vi "浮标电源管理UI.vi"() -> ()   [LabVIEW 2016, in "环境动力监测库.lvlib" / "浮标电源管理.lvlib"]
uses:
  <vilib>/Utility/miscctls.llb/LVPointTypeDef.ctl
  <vilib>/Utility/config.llb/NI_LVConfig.lvlib
  <vilib>/ptbypt/NI_PtbyPt.lvlib
panel:
  in  "控制对象":enum16{"所有辅助设备", "气象电源", "视频电源"}(ring)=enum."视频电源"
  in  "辅助电源控制类型":enum16{"定时控制", "电压控制"}(ring)
  in  "辅助设备电源关闭时间":u16(ring)=12 items=["00H", "01H", "02H", "03H", "04H", "05H", "06H", "07H", "08H", "09H", "10H", "11H", "12H", "13H", "14H", "15H", "16H", "17H", "18H", "19H", "20H", "21H", "22H", "23H"]
  in  "辅助设备电源开启时间":u16(ring)=12 items=["00H", "01H", "02H", "03H", "04H", "05H", "06H", "07H", "08H", "09H", "10H", "11H", "12H", "13H", "14H", "15H", "16H", "17H", "18H", "19H", "20H", "21H", "22H", "23H"]
  in  "开启辅助电源控制":bool
  in  "辅助设备电源开启电压 V":dbl=13.0
  in  "辅助设备电源关闭电压 V":dbl=12.0
  in  "视频电源":bool
  in  "气象电源":bool
  in  "总磷总氮电源":bool
  in  "氨氮电源":bool
  in  "多参数电源":bool
  in  "IO模块启用":bool
  in  "IO串口":refnum<visa-resource-name>
  in  "串口启用":bool
  out "电压报警":bool
  in  "低压报警解除阈值 V":dbl=50.0
  in  "低压报警阈值 V":dbl=50.0
  out "当前电压":dbl=21.0 format="%.2f V"
  out "通讯状态":bool
  # "仪器电源管理"
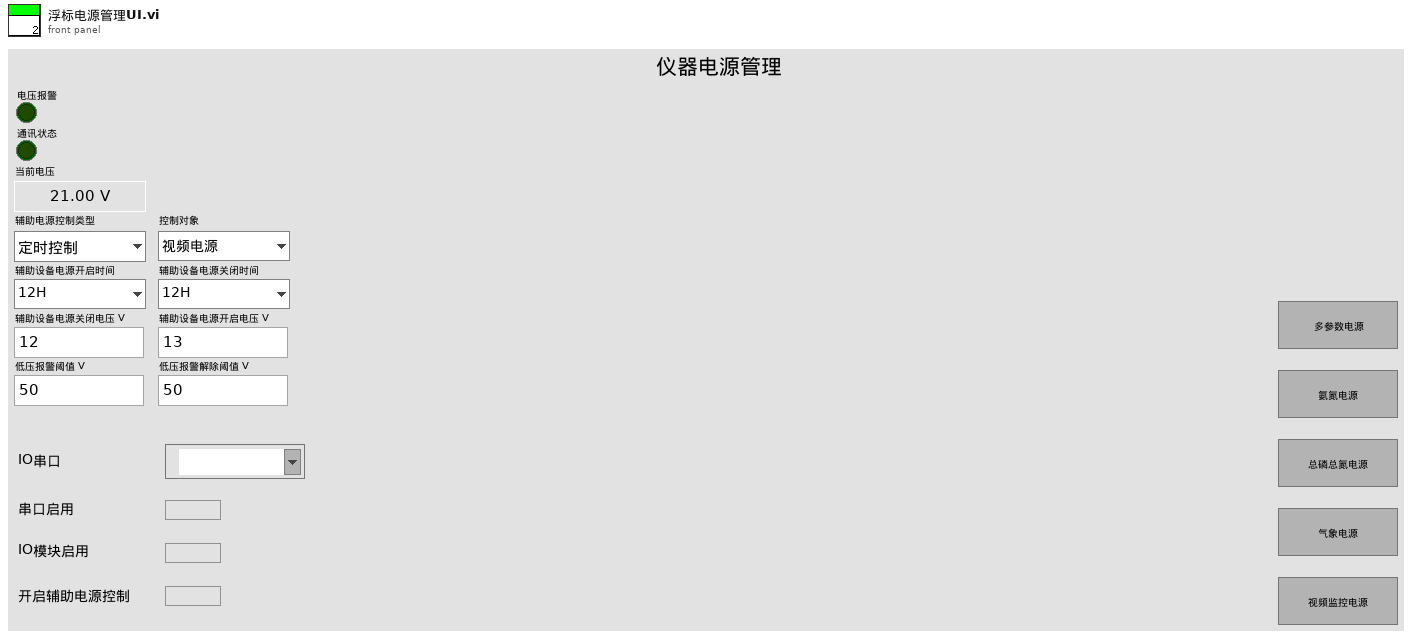
[diagram p1: front panel]
types:
  T1 = typedef "LVPointTypeDef.ctl" = cluster{"Horizontal":i16, "Vertical":i16}
  T2 = cluster{"AD0":dbl, "AD1":dbl, "AD2":dbl, "AD3":dbl, "AD4":dbl, "AD5":dbl, "AD6":dbl, "AD7":dbl}
  T3 = cluster{"低压报警阈值 V":dbl, "低压报警解除阈值 V":dbl, "高温报警阈值 ℃":dbl, "高温报警解除阈值 ℃":dbl, "湿度报警阈值 %":dbl, "湿度报警解除阈值 %":dbl}
  T4 = typedef "LVDateTimeRec.ctl" = cluster{"秒数的小数部分":dbl, "秒":i32, "分":i32, "时":i32, "日":i32, "月":i32, "年":i32, "天数（周）":i32, "天数（年）":i32, "DST":i32}
  T5 = cluster{"时间标识":timestamp, "设备":string, "报警信息":string}
  T6 = typedef "NI_LVConfig.lvlib/Config Data RefNum.ctl" = refnum<k1>
  T7 = enum8{"Enabled", "Disabled", "Disabled and Grayed Out"}
  T8 = cluster{"Registers[0]":u16, "Registers[1]":u16, "Registers[2]":u16, "Registers[3]":u16, "Registers[4]":u16, "Registers[5]":u16, "Registers[6]":u16, "Registers[7]":u16}
  T9 = cluster{"网络状态":bool, "电源管理":cluster{"电源管理":bool, "氨氮电源":bool, "总磷电源":bool, "总氮电源":bool, "多参数电源":bool, "CODMn电源":bool, "CODCr电源":bool, "灯带电源":bool, "照明电源":bool}, "北斗-GPS":cluster{"北斗":cluster{"经度:":sgl, "纬度:":sgl, "北斗监测":bool}, "GPS":cluster{"经度:":sgl, "纬度: ":sgl, "GPS监测":bool}}}
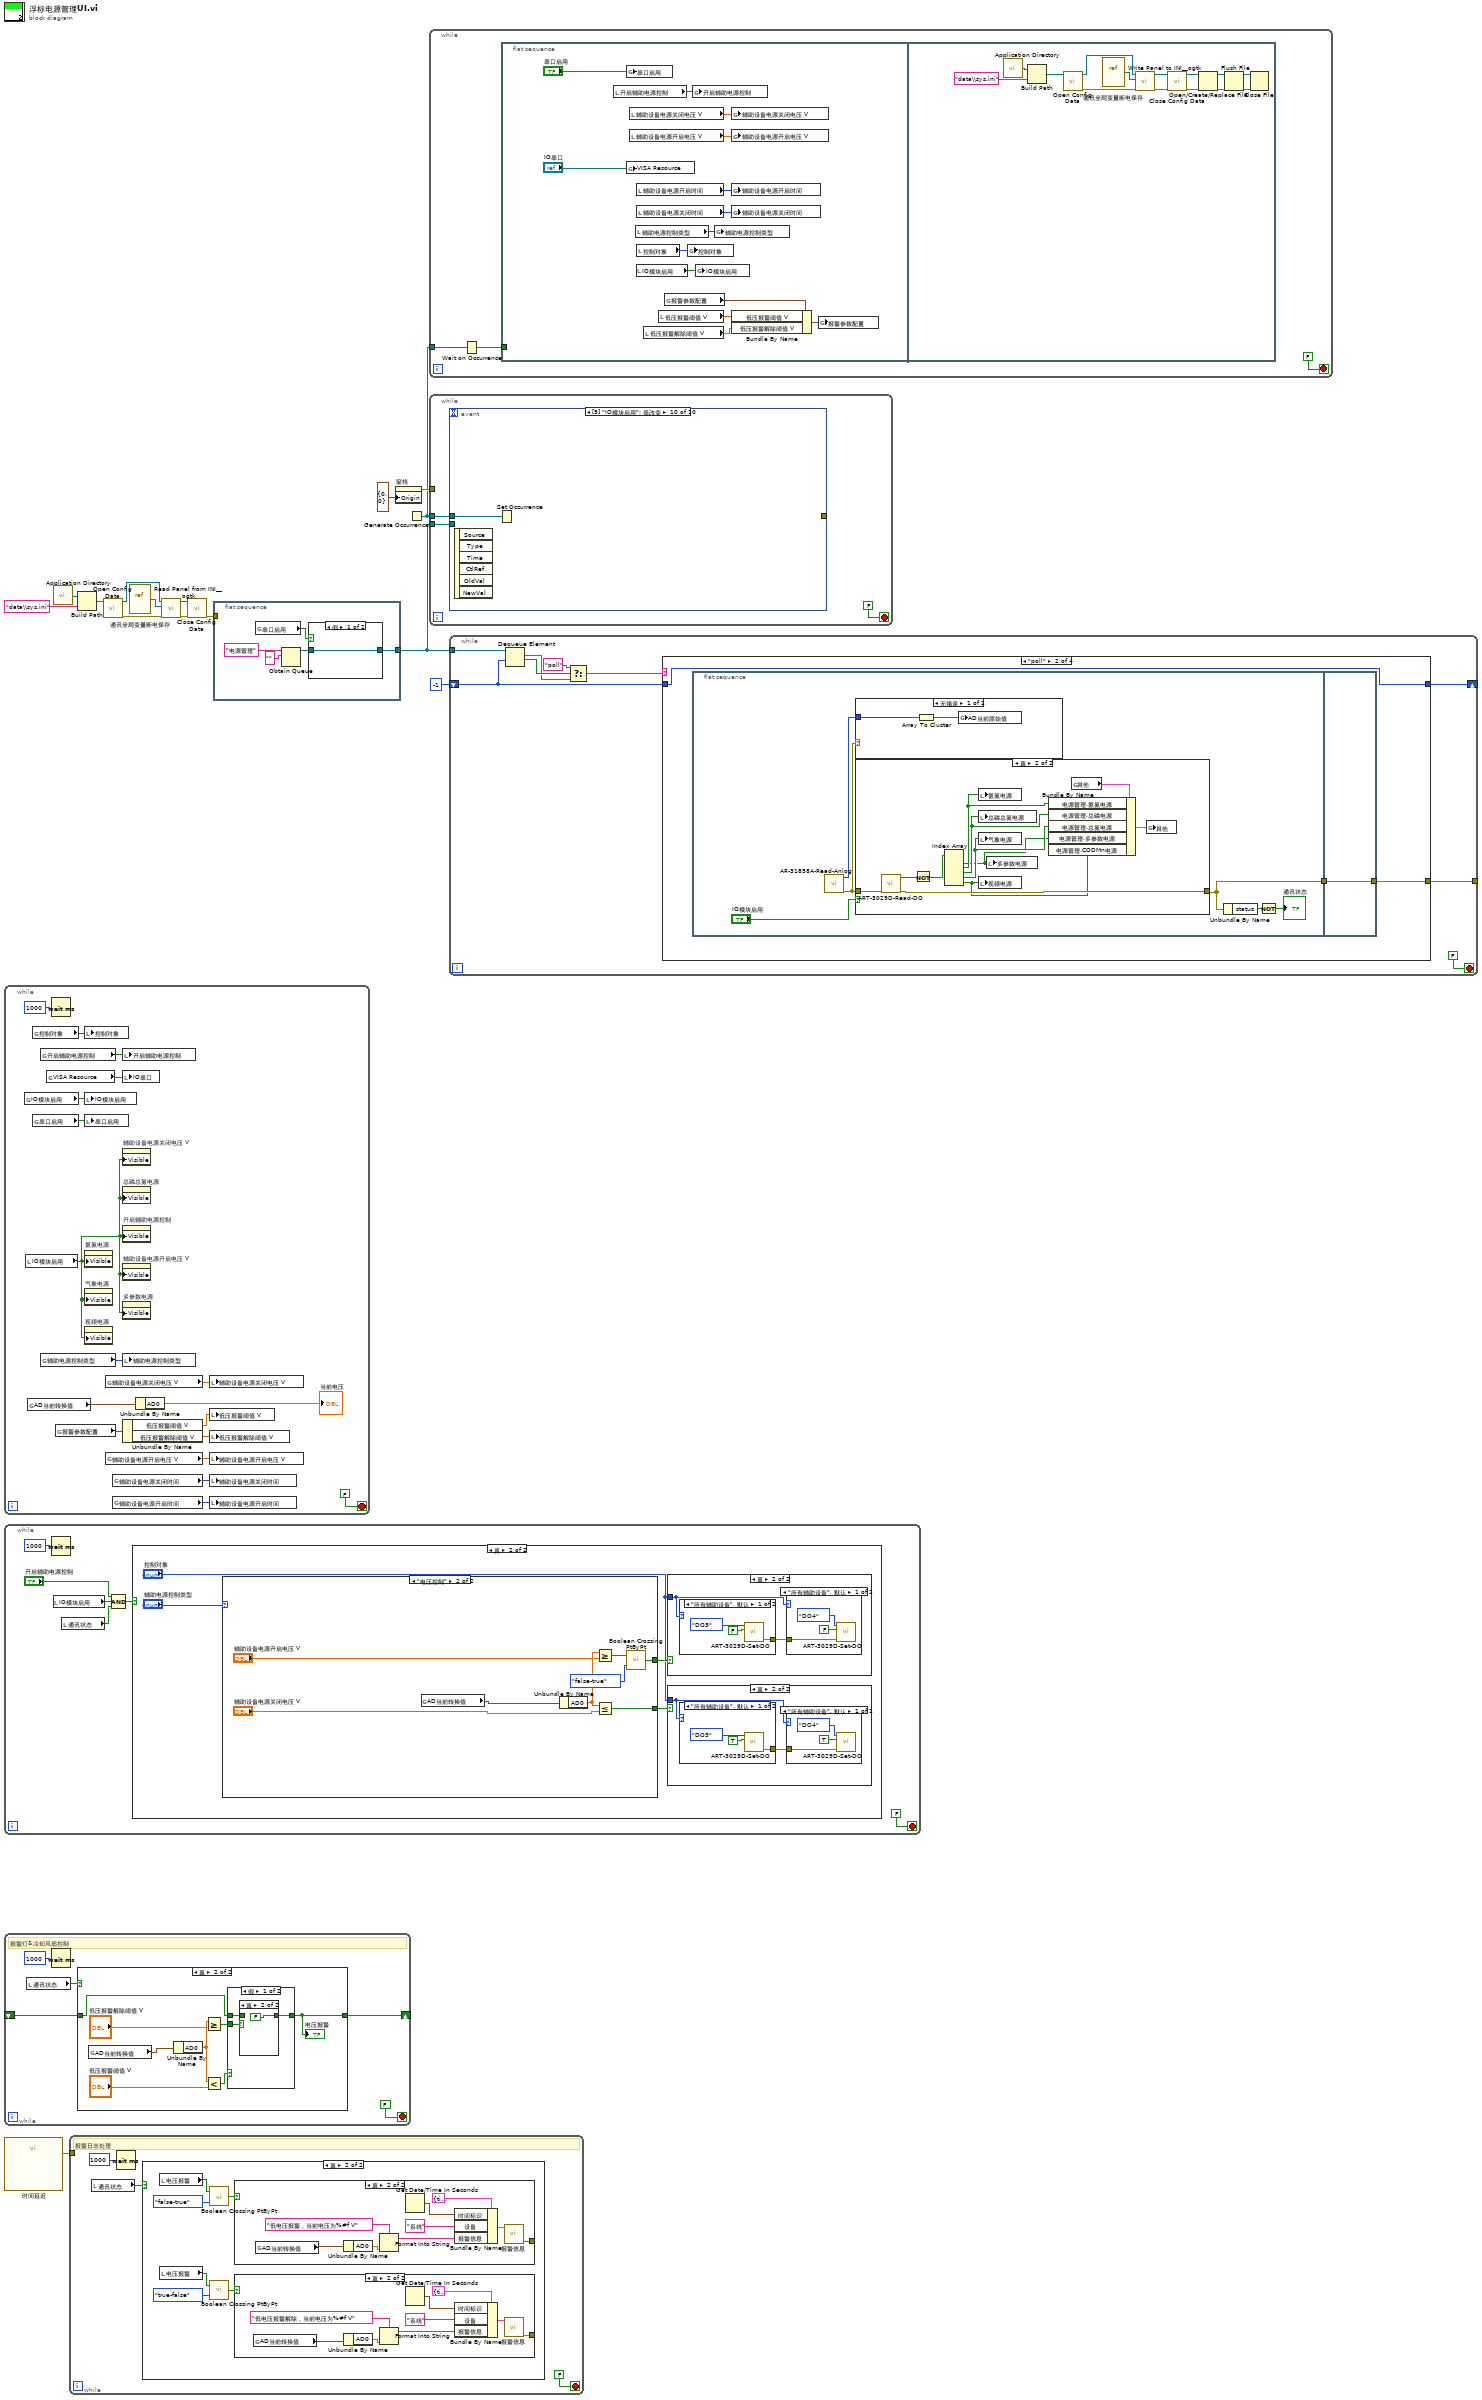
[diagram p0: block diagram]
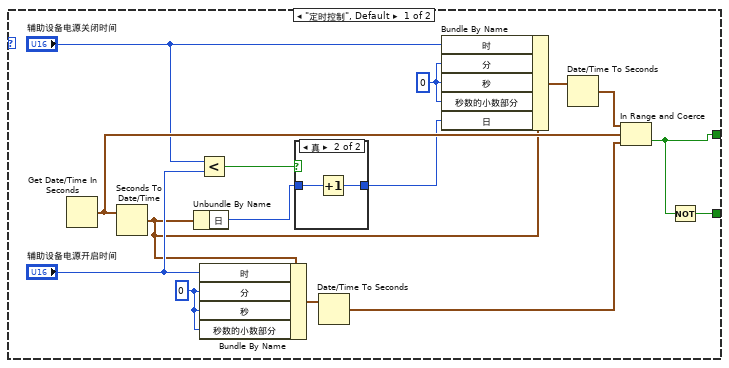
[diagram p6: hidden frame]
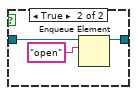
[diagram p11: hidden frame]
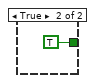
[diagram p17: hidden frame]
diagram:
  n1 = while {
    stop <- FALSE stop-if-true
    n2 = global read "通讯全局变量断电保存.vi" "IO模块启用"() -> (w25:bool)
    n3 = local read "IO模块启用"() -> (w22:bool)
    n4 = global read "断电保存全局变量.vi" "AD当前转换值"() -> (w16:T2)
    n5 = global read "通讯全局变量断电保存.vi" "控制对象"() -> (w17:enum16{"所有辅助设备", "气象电源", "视频电源"})
    n6 = global read "通讯全局变量断电保存.vi" "串口启用"() -> (w27:bool)
    n7 = global read "通讯全局变量断电保存.vi" "开启辅助电源控制"() -> (w21:bool)
    n8 = global read "通讯全局变量断电保存.vi" "辅助电源控制类型"() -> (w20:enum16{"定时控制", "电压控制"})
    n9 = global read "通讯全局变量断电保存.vi" "VISA Resource"() -> (w26:refnum<visa-resource-name>)
    n10 = Wait (ms)(milliseconds to wait=u32 1000 ("等待时间（毫秒）")) -> ()  [unwired: 1 out]
    n11 = global read "通讯全局变量断电保存.vi" "报警参数配置"() -> (w32:T3)
    n12 = local write "控制对象"(w17) -> ()
    n13 = local write "IO模块启用"(w25) -> ()
    n14 = local write "串口启用"(w27) -> ()
    n15 = property on="氨氮电源" class="Bool (严格)"("Visible"=w22) -> ()  [unwired: 2 in, 2 out]
    n16 = property on="气象电源" class="Bool (严格)"("Visible"=w22) -> ()  [unwired: 2 in, 2 out]
    n17 = property on="视频电源" class="Bool (严格)"("Visible"=w22) -> ()  [unwired: 2 in, 2 out]
    n18 = global read "通讯全局变量断电保存.vi" "辅助设备电源关闭电压 V"() -> (w24:dbl)
    n19 = global read "通讯全局变量断电保存.vi" "辅助设备电源开启电压 V"() -> (w23:dbl)
    n20 = global read "通讯全局变量断电保存.vi" "辅助设备电源关闭时间"() -> (w19:u16)
    n21 = global read "通讯全局变量断电保存.vi" "辅助设备电源开启时间"() -> (w18:u16)
    n22 = local write "开启辅助电源控制"(w21) -> ()
    n23 = local write "IO串口"(w26) -> ()
    n24 = property on="辅助设备电源关闭电压 V" class="DigNum (严格)"("Visible"=w22) -> ()  [unwired: 2 in, 2 out]
    n25 = property on="总磷总氮电源" class="Bool (严格)"("Visible"=w22) -> ()  [unwired: 2 in, 2 out]
    n26 = property on="开启辅助电源控制" class="Bool (严格)"("Visible"=w22) -> ()  [unwired: 2 in, 2 out]
    n27 = property on="辅助设备电源开启电压 V" class="DigNum (严格)"("Visible"=w22) -> ()  [unwired: 2 in, 2 out]
    n28 = property on="多参数电源" class="Bool (严格)"("Visible"=w22) -> ()  [unwired: 2 in, 2 out]
    n29 = local write "辅助电源控制类型"(w20) -> ()
    n30 = Unbundle By Name(w32) -> ("低压报警阈值 V"=w30:dbl, "低压报警解除阈值 V"=w29:dbl)
    n31 = Unbundle By Name(w16) -> ("AD0"=→"当前电压":dbl)
    n32 = local write "辅助设备电源关闭电压 V"(w24) -> ()
    n33 = local write "低压报警阈值 V"(w30) -> ()
    n34 = local write "低压报警解除阈值 V"(w29) -> ()
    n35 = local write "辅助设备电源开启电压 V"(w23) -> ()
    n36 = local write "辅助设备电源关闭时间"(w19) -> ()
    n37 = local write "辅助设备电源开启时间"(w18) -> ()
  }
  n38 = while {
    stop <- FALSE stop-if-true
    n39 = Wait (ms)(milliseconds to wait=u32 1000 ("等待时间（毫秒）")) -> ()  [unwired: 1 out]
    n40 = local read "IO模块启用"() -> (w36:bool)
    n41 = local read "通讯状态"() -> (w37:bool)
    n42 = Compound Arithmetic op=AND ("复合运算")("开启辅助电源控制", w36, w37) -> (w34:bool)
    n43 = case shown="真" w34 {
      frame False {
      }
      frame True {
        n44 = case shown="\"电压控制\"" "辅助电源控制类型" {
          tunnel: [w53 w72] -> w41
          tunnel: [w52 w71] -> w43
          frame "定时控制", Default {
            w55 = 0
            w54 = 0
            n45 = Get Date/Time In Seconds() -> (seconds since 1Jan1904=w66:timestamp)
            n46 = Seconds To Date/Time(time stamp (now)=w66) -> (date time rec=w60:T4)  [unwired: 1 in]
            n47 = Unbundle By Name(w60) -> ("日"=w61:i32)
            n48 = Less?(x="辅助设备电源关闭时间", y="辅助设备电源开启时间") -> (x < y?=w63:bool)
            n49 = Bundle By Name(cluster=w60, "时"="辅助设备电源开启时间", "分"=w54, "秒"=w54, "秒数的小数部分"=w54) -> (w56:T4)
            n50 = case shown="真" w63 {
              tunnel: w61 -> [w67 w69]
              tunnel: [w67 w68] -> w62
              frame False {
              }
              frame True {
                n51 = Increment(x=w69) -> (x+1=w68:i32)
              }
            }
            n52 = Date/Time To Seconds(2:w56) -> (0:w59:timestamp)  [unwired: 1 in]
            n53 = Bundle By Name(cluster=w60, "时"="辅助设备电源关闭时间", "分"=w55, "秒"=w55, "秒数的小数部分"=w55, "日"=w62) -> (w57:T4)
            n54 = Date/Time To Seconds(2:w57) -> (0:w58:timestamp)  [unwired: 1 in]
            n55 = In Range and Coerce(upper limit=w58, x=w66, lower limit=w59) -> (In Range?=w53:bool)  [unwired: 1 out]
            n56 = Not(x=w53) -> (.not. x?=w52:bool)
          }
          frame "电压控制" {
            n57 = global read "断电保存全局变量.vi" "AD当前转换值"() -> (w70:T2)
            n58 = Unbundle By Name(w70) -> ("AD0"=w76:dbl)
            n59 = Greater Or Equal?(x=w76, y="辅助设备电源开启电压 V") -> (x >= y?=w73:bool)
            n60 = Less Or Equal?(x=w76, y="辅助设备电源关闭电压 V") -> (x <= y?=w71:bool)
            n61 = call <vilib>:"Boolean Crossing PtByPt.vi"("direction"=enum16{"either", "false-true", "true-false"}."false-true", "input"=w73) -> ("crossing"=w72:bool)  [unwired: 1 in]
          }
        }
        n62 = case shown="真" w41 {
          tunnel: "控制对象" -> [_ w44]
          frame False {
          }
          frame True {
            n63 = case shown="\"所有辅助设备\", 默认" w44 {
              tunnel: [w50 _] -> w45
              frame "所有辅助设备", Default {
                n64 = call "ART-3029D-Set-DO.vi"("value"=FALSE, "DI"=enum16{"DO0", "DO1", "DO2", "DO3", "DO4"}."DO3") -> ("error out"=w50:errorcluster)  [unwired: 9 in]
              }
              frame "视频电源" {
              }
            }
            n65 = case shown="\"所有辅助设备\", 默认" w44 {
              tunnel: w45 -> [w48 _]
              frame "所有辅助设备", Default {
                n66 = call "ART-3029D-Set-DO.vi"("error in (no error)"=w48, "value"=FALSE, "DI"=enum16{"DO0", "DO1", "DO2", "DO3", "DO4"}."DO4") -> ()  [unwired: 8 in, 1 out]
              }
              frame "气象电源" {
              }
            }
          }
        }
        n67 = case shown="真" w43 {
          tunnel: "控制对象" -> [_ w78]
          frame False {
          }
          frame True {
            n68 = case shown="\"所有辅助设备\", 默认" w78 {
              tunnel: [w84 _] -> w79
              frame "所有辅助设备", Default {
                n69 = call "ART-3029D-Set-DO.vi"("value"=TRUE, "DI"=enum16{"DO0", "DO1", "DO2", "DO3", "DO4"}."DO3") -> ("error out"=w84:errorcluster)  [unwired: 9 in]
              }
              frame "视频电源" {
              }
            }
            n70 = case shown="\"所有辅助设备\", 默认" w78 {
              tunnel: w79 -> [w82 _]
              frame "所有辅助设备", Default {
                n71 = call "ART-3029D-Set-DO.vi"("error in (no error)"=w82, "value"=TRUE, "DI"=enum16{"DO0", "DO1", "DO2", "DO3", "DO4"}."DO4") -> ()  [unwired: 8 in, 1 out]
              }
              frame "气象电源" {
              }
            }
          }
        }
      }
    }
  }
  n72 = while {
    shift-right: [w87] -> _
    shift-left: _ -> [w86]
    stop <- FALSE stop-if-true
    # "报警灯&冷却风扇控制"
    n73 = local read "通讯状态"() -> (w90:bool)
    n74 = Wait (ms)(milliseconds to wait=u32 1000 ("等待时间（毫秒）")) -> ()  [unwired: 1 out]
    n75 = case shown="真" w90 {
      tunnel: [_ w92] -> w87
      tunnel: w86 -> [_ w94]
      frame False {
      }
      frame True {
        n76 = global read "断电保存全局变量.vi" "AD当前转换值"() -> (w91:T2)
        n77 = Unbundle By Name(w91) -> ("AD0"=w96:dbl)
        n78 = Greater Or Equal?(x=w96, y="低压报警解除阈值 V") -> (x >= y?=w95:bool)
        n79 = Less?(x=w96, y="低压报警阈值 V") -> (x < y?=w97:bool)
        n80 = case shown="假" w97 {
          tunnel: [w99 TRUE] -> w92
          tunnel: w94 -> [w100 _]
          tunnel: w95 -> [w101 _]
          frame False {
            n81 = case shown="真" w101 {
              tunnel: [w102 FALSE] -> w99
              tunnel: w100 -> [w102 _]
              frame False {
              }
              frame True {
              }
            }
          }
          frame True {
          }
        }
        "电压报警" <- w92
      }
    }
  }
  n82 = call "时间延迟"() -> ("error out"=w5:errorcluster)  [unwired: 11 in]
  n83 = call <vilib>:"Application Directory.vi"() -> ("Application Directory"=w7:path)
  n84 = while {
    tunnel: w5 -> [_]
    stop <- FALSE stop-if-true
    # "报警日志处理"
    n85 = local read "通讯状态"() -> (w106:bool)
    n86 = Wait (ms)(milliseconds to wait=u32 1000 ("等待时间（毫秒）")) -> ()  [unwired: 1 out]
    n87 = case shown="真" w106 {
      frame False {
      }
      frame True {
        n88 = local read "电压报警"() -> (w109:bool)
        n89 = local read "电压报警"() -> (w111:bool)
        n90 = call <vilib>:"Boolean Crossing PtByPt.vi"("direction"=enum16{"either", "false-true", "true-false"}."false-true", "input"=w109) -> ("crossing"=w108:bool)  [unwired: 1 in]
        n91 = call <vilib>:"Boolean Crossing PtByPt.vi"("direction"=enum16{"either", "false-true", "true-false"}."true-false", "input"=w111) -> ("crossing"=w112:bool)  [unwired: 1 in]
        n92 = case shown="真" w108 {
          tunnel: [_ w126] -> _
          frame False {
          }
          frame True {
            n93 = global read "断电保存全局变量.vi" "AD当前转换值"() -> (w123:T2)
            n94 = Unbundle By Name(w123) -> ("AD0"=w125:dbl)
            n95 = Format Into String(format string="低电压报警，当前电压为%#f V" ("报警信息"), w125) -> (resulting string=w124:string)  [unwired: 2 in, 1 out]
            n96 = Get Date/Time In Seconds() -> (seconds since 1Jan1904=w131:timestamp)
            n97 = Bundle By Name(cluster=T5 {"时间标识"=timestamp(0 s since 1904-01-01), "设备"="", "报警信息"=""} ("data in"), "时间标识"=w131, "设备"="系统", "报警信息"=w124) -> (w129:T5)
            n98 = call "报警信息.vi"("data in"=w129) -> ("error out"=w126:errorcluster)  [unwired: 10 in]
          }
        }
        n99 = case shown="真" w112 {
          tunnel: [_ w117] -> _
          frame False {
          }
          frame True {
            n100 = global read "断电保存全局变量.vi" "AD当前转换值"() -> (w114:T2)
            n101 = Unbundle By Name(w114) -> ("AD0"=w116:dbl)
            n102 = Format Into String(format string="低电压报警解除，当前电压为%#f V" ("报警信息"), w116) -> (resulting string=w115:string)  [unwired: 2 in, 1 out]
            n103 = Get Date/Time In Seconds() -> (seconds since 1Jan1904=w122:timestamp)
            n104 = Bundle By Name(cluster=T5 {"时间标识"=timestamp(0 s since 1904-01-01), "设备"="", "报警信息"=""} ("data in"), "时间标识"=w122, "设备"="系统", "报警信息"=w115) -> (w120:T5)
            n105 = call "报警信息.vi"("data in"=w120) -> ("error out"=w117:errorcluster)  [unwired: 10 in]
          }
        }
      }
    }
  }
  n106 = Build Path(base path=w7, name or relative path="data\\sys.ini" ("名称或相对路径")) -> (appended path=w9:path)
  n107 = call <vilib>:"Open Config Data.vi"("configuration file path"=w9) -> ("error out"=w13:errorcluster, "refnum"=w10:T6)  [unwired: 8 in, 1 out]
  n108 = vi-ref "通讯全局变量断电保存.vi"() -> (w11:refnum<vi>)
  n109 = call <userlib>:"Read Panel from INI__ogtk.vi"("error in (no error)"=w13, "VI ref"=w11, "refnum"=w10) -> ("error out"=w6:errorcluster, "refnum out"=w12:T6)  [unwired: 7 in]
  n110 = call <vilib>:"Close Config Data.vi"("error in (no error)"=w6, "refnum"=w12) -> ("error out"=w1:errorcluster)  [unwired: 8 in, 1 out]
  n111 = flat-sequence {
    tunnel: [w133] -> w4
    tunnel: w1 -> [_]
    frame #0 {
      n112 = global read "通讯全局变量断电保存.vi" "串口启用"() -> (w132:bool)
      n113 = Obtain Queue(name (unnamed)="电源管理" ("名称（未命名）"), element data type="") -> (queue out=w134:refnum<queue>)  [unwired: 3 in, 2 out]
      n114 = case shown="假" w132 {
        tunnel: w134 -> [w137 w140]
        tunnel: [w137 w138] -> w133
        frame False {
        }
        frame True {
          n115 = Enqueue Element(queue=w140, element="open" ("元素")) -> (queue out=w138:refnum<queue>)  [unwired: 2 in, 2 out]
        }
      }
    }
  }
  n116 = property on="窗格" class="Pane"("Origin"=T1 {"Horizontal"=0, "Vertical"=0} ("原点")) -> (error out=w14:errorcluster)  [unwired: 2 in, 1 out]
  n117 = Generate Occurrence() -> (w2:refnum<k4>)
  n118 = while {
    tunnel: w2 -> [w142]
    stop <- FALSE stop-if-true
    n119 = Wait on Occurrence(2:w142) -> (0:w141:bool)  [unwired: 2 in]
    n120 = flat-sequence {
      tunnel: w141 -> [_]
      frame #0 {
        n121 = local read "开启辅助电源控制"() -> (w148:bool)
        n122 = global write "通讯全局变量断电保存.vi" "串口启用"("串口启用") -> ()
        n123 = global write "通讯全局变量断电保存.vi" "VISA Resource"("IO串口") -> ()
        n124 = local read "辅助设备电源关闭电压 V"() -> (w150:dbl)
        n125 = local read "辅助设备电源开启电压 V"() -> (w149:dbl)
        n126 = local read "辅助电源控制类型"() -> (w146:enum16{"定时控制", "电压控制"})
        n127 = local read "IO模块启用"() -> (w151:bool)
        n128 = local read "辅助设备电源开启时间"() -> (w147:u16)
        n129 = local read "辅助设备电源关闭时间"() -> (w145:u16)
        n130 = local read "控制对象"() -> (w144:enum16{"所有辅助设备", "气象电源", "视频电源"})
        n131 = local read "低压报警解除阈值 V"() -> (w154:dbl)
        n132 = local read "低压报警阈值 V"() -> (w155:dbl)
        n133 = global read "通讯全局变量断电保存.vi" "报警参数配置"() -> (w157:T3)
        n134 = global write "通讯全局变量断电保存.vi" "控制对象"(w144) -> ()
        n135 = global write "通讯全局变量断电保存.vi" "开启辅助电源控制"(w148) -> ()
        n136 = global write "通讯全局变量断电保存.vi" "IO模块启用"(w151) -> ()
        n137 = global write "通讯全局变量断电保存.vi" "辅助电源控制类型"(w146) -> ()
        n138 = global write "通讯全局变量断电保存.vi" "辅助设备电源关闭电压 V"(w150) -> ()
        n139 = global write "通讯全局变量断电保存.vi" "辅助设备电源开启电压 V"(w149) -> ()
        n140 = global write "通讯全局变量断电保存.vi" "辅助设备电源开启时间"(w147) -> ()
        n141 = global write "通讯全局变量断电保存.vi" "辅助设备电源关闭时间"(w145) -> ()
        n142 = Bundle By Name(cluster=w157, "低压报警阈值 V"=w155, "低压报警解除阈值 V"=w154) -> (w156:T3)
        n143 = global write "通讯全局变量断电保存.vi" "报警参数配置"(w156) -> ()
      }
      frame #1 {
        n144 = call <vilib>:"Application Directory.vi"() -> ("Application Directory"=w171:path)
        n145 = Build Path(base path=w171, name or relative path="data\\sys.ini" ("名称或相对路径")) -> (appended path=w169:path)
        n146 = call <vilib>:"Open Config Data.vi"("configuration file path"=w169) -> ("error out"=w165:errorcluster, "refnum"=w168:T6)  [unwired: 8 in, 1 out]
        n147 = vi-ref "通讯全局变量断电保存.vi"() -> (w167:refnum<vi>)
        n148 = call <userlib>:"Write Panel to INI__ogtk.vi"("error in (no error)"=w165, "VI ref"=w167, "refnum"=w168) -> ("error out"=w164:errorcluster, "refnum out"=w166:T6)  [unwired: 7 in]
        n149 = call <vilib>:"Close Config Data.vi"("error in (no error)"=w164, "refnum"=w166) -> ("error out"=w159:errorcluster, "file path"=w158:path)  [unwired: 8 in]
        n150 = Open/Create/Replace File(file path (use dialog)=w158, error in=w159) -> (refnum out=w162:refnum<file>, error out=w163:errorcluster)  [unwired: 4 in, 1 out]
        n151 = Flush File(refnum=w162, error in=w163) -> (refnum out=w161:refnum<file>, error out=w160:errorcluster)
        n152 = Close File(refnum=w161, error in=w160) -> ()  [unwired: 2 out]
      }
    }
  }
  n153 = while {
    tunnel: w14 -> [_]
    tunnel: w4 -> [w173]
    tunnel: w2 -> [w172]
    stop <- FALSE stop-if-true
    n154 = event shown="[9] \"IO模块启用\": 值改变" {
      selector: _ -> [_ _ _ _ _ _ _ _ _ _]
      dyn-events: _ -> [_ _ _ _ _ _ _ _ _ _]
      timeout: _ -> [_ _ _ _ _ _ _ _ _ _]
      tunnel: w173 -> [_ _ _ _ _ _ _ _ w198 _]
      tunnel: w172 -> [_ _ _ _ _ _ _ w194 w200 w201]
      tunnel: [_ w177 w180 w183 w186 w189 _ _ _ _] -> _
      event Timeout {
        n155 = event-data() -> ()  [unwired: 1 in, 3 out]
      }
      event "多参数电源": Value Change {
        n156 = event-data() -> ("OldVal"=w175:bool)  [unwired: 1 in, 5 out]
        n157 = call "ART-3029D-Set-DO.vi"("value"=w175, "DI"=enum16{"DO0", "DO1", "DO2", "DO3", "DO4"}."DO0") -> ("error out"=w177:errorcluster)  [unwired: 9 in]
      }
      event "氨氮电源": Value Change {
        n158 = event-data() -> ("OldVal"=w178:bool)  [unwired: 1 in, 5 out]
        n159 = call "ART-3029D-Set-DO.vi"("value"=w178, "DI"=enum16{"DO0", "DO1", "DO2", "DO3", "DO4"}."DO1") -> ("error out"=w180:errorcluster)  [unwired: 9 in]
      }
      event "总磷总氮电源": Value Change {
        n160 = event-data() -> ("OldVal"=w181:bool)  [unwired: 1 in, 5 out]
        n161 = call "ART-3029D-Set-DO.vi"("value"=w181, "DI"=enum16{"DO0", "DO1", "DO2", "DO3", "DO4"}."DO2") -> ("error out"=w183:errorcluster)  [unwired: 9 in]
      }
      event "气象电源": Value Change {
        n162 = event-data() -> ("OldVal"=w184:bool)  [unwired: 1 in, 5 out]
        n163 = call "ART-3029D-Set-DO.vi"("value"=w184, "DI"=enum16{"DO0", "DO1", "DO2", "DO3", "DO4"}."DO3") -> ("error out"=w186:errorcluster)  [unwired: 9 in]
      }
      event "视频电源": Value Change {
        n164 = event-data() -> ("OldVal"=w187:bool)  [unwired: 1 in, 5 out]
        n165 = call "ART-3029D-Set-DO.vi"("value"=w187, "DI"=enum16{"DO0", "DO1", "DO2", "DO3", "DO4"}."DO4") -> ("error out"=w189:errorcluster)  [unwired: 9 in]
      }
      event "低压报警阈值 V", "低压报警解除阈值 V", "辅助设备电源关闭电压 V", "辅助设备电源开启电压 V": Mouse Down {
        n166 = event-data() -> ("CtlRef"=w193:refnum<vi>)  [unwired: 1 in, 5 out]
        n167 = property class="DigNum (严格)"(reference=w193) -> (reference out=w191:refnum<vi>, "Value"=w192:dbl)  [unwired: 1 in, 1 out]
        n168 = call "数字键盘.vi"("OldNumber"=w192) -> ("NewNumber"=w190:sgl)
        n169 = property class="DigNum (严格)"(reference=w191, "Val(Sgnl)"=w190) -> ()  [unwired: 1 in, 2 out]
      }
      event "IO串口", "低压报警阈值 V", "低压报警解除阈值 V", "辅助设备电源关闭电压 V", "辅助设备电源开启电压 V", "开启辅助电源控制", "辅助设备电源开启时间", "辅助设备电源关闭时间", "辅助电源控制类型", "控制对象": Value Change {
        n170 = event-data() -> ()  [unwired: 1 in, 6 out]
        n171 = Set Occurrence(w194) -> ()
      }
      event "串口启用": Value Change {
        n172 = event-data() -> ("NewVal"=w199:bool)  [unwired: 1 in]
        n173 = Set Occurrence(w200) -> ()
        n174 = Select(t="open", s=w199, f="close") -> (s? t:f=w196:string)
        n175 = Enqueue Element(queue=w198, element=w196) -> ()  [unwired: 2 in, 3 out]
      }
      event "IO模块启用": Value Change {
        n176 = event-data() -> ()  [unwired: 1 in, 6 out]
        n177 = Set Occurrence(w201) -> ()
      }
    }
  }
  n178 = while {
    tunnel: w4 -> [w210]
    tunnel: [w204] -> _
    shift-right: [w202] -> _
    shift-left: -1 ("超时毫秒(-1)") -> [w203]
    stop <- FALSE stop-if-true
    n179 = Dequeue Element(queue=w210, timeout in ms (-1)=w203) -> (element=w207:string, timed out?=w209:bool)  [unwired: 1 in, 2 out]
    n180 = Select(t="poll" ("元素"), s=w209, f=w207) -> (s? t:f=w206:string)
    n181 = case shown="\"poll\"" w206 {
      tunnel: [_ w214 w237 w243] -> w204
      tunnel: w203 -> [w211 w212 _ _]
      tunnel: [w211 w212 1000 ("超时毫秒(-1)") -1 ("超时毫秒(-1)")] -> w202
      frame Default {
      }
      frame "poll" {
        n182 = flat-sequence {
          tunnel: [w215] -> w213
          tunnel: [w235] -> w214
          tunnel: w213 -> [w235]
          frame #0 {
            n183 = call "AR-31858A-Read-Anlog.vi"() -> ("error out"=w217:errorcluster, "Registers"=w218:u16[])  [unwired: 10 in]
            n184 = case shown="无错误" w217 {
              tunnel: w218 -> [w234 _]
              frame No Error {
                n185 = Array To Cluster(array=w234) -> (cluster=w233:T8)
                n186 = global write "断电保存全局变量.vi" "AD当前原始值"(w233) -> ()
              }
              frame Error {
              }
            }
            n187 = case shown="真" "IO模块启用" {
              tunnel: w217 -> [w221 w232]
              tunnel: [w221 w231] -> w215
              frame False {
              }
              frame True {
                n188 = call "ART-3029D-Read-DO.vi"("error in (no error)"=w232) -> ("error out"=w231:errorcluster, "Coils"=w230:bool[])  [unwired: 9 in]
                n189 = Not(x=w230) -> (.not. x?=w229:bool[])
                n190 = Index Array(array=w229) -> (element #1=w223:bool, element #2=w226:bool, element #3=w225:bool, element #4=w224:bool, element #5=w222:bool)  [unwired: 5 in]
                n191 = local write "氨氮电源"(w226) -> ()
                n192 = local write "总磷总氮电源"(w225) -> ()
                n193 = local write "气象电源"(w224) -> ()
                n194 = local write "视频电源"(w222) -> ()
                n195 = local write "多参数电源"(w223) -> ()
                n196 = global read "内部交互全局变量.vi" "其他"() -> (w227:T9)
                n197 = Bundle By Name(cluster=w227, "电源管理.氨氮电源"=w226, "电源管理.总磷电源"=w225, "电源管理.总氮电源"=w224, "电源管理.多参数电源"=w223, "电源管理.CODMn电源"=w222) -> (w228:T9)
                n198 = global write "内部交互全局变量.vi" "其他"(w228) -> ()
              }
            }
            n199 = Unbundle By Name(w215) -> ("status"=w219:bool)
            n200 = Not(x=w219) -> (.not. x?=→"通讯状态":bool)
          }
          frame #1 {
          }
        }
      }
      frame "open" {
        n201 = local write "通讯状态"(FALSE ("通讯状态")) -> ()
        n202 = call "open MB.vi"() -> ("error out"=w237:errorcluster)  [unwired: 11 in]
        n203 = case shown="无错误" w237 {
          tunnel: [T7."Disabled and Grayed Out" ("禁用") T7."Enabled" ("禁用")] -> w236
          frame No Error {
          }
          frame Error {
            n204 = global write "通讯全局变量断电保存.vi" "串口启用"(FALSE ("串口启用")) -> ()
          }
        }
        n205 = property on="IO串口" class="VISAName"("DisabledEnum"=w236) -> ()  [unwired: 2 in, 2 out]
      }
      frame "close" {
        n206 = call "close MB.vi"() -> ("error out"=w243:errorcluster)  [unwired: 11 in]
        n207 = case shown="无错误" w243 {
          frame No Error {
            n208 = property on="IO串口" class="VISAName"("DisabledEnum"=T7."Enabled" ("禁用")) -> ()  [unwired: 2 in, 2 out]
          }
          frame Error {
          }
        }
      }
    }
  }
